vi "Stop Core.vi"(10 "final error code":i32, 11 "tWorkerTCPConnection in":refnum<class "tWorkerTCPConnection.lvclass">) -> (3 "tWorkerTCPConnection out":refnum<class "tWorkerTCPConnection.lvclass">)   [LabVIEW 2013, in "tWorkerTCPConnection.lvlib" / "tWorkerTCPConnection.lvclass"]
doc: "(<B>Filename</B>: Actor Framework.lvlib:Actor.lvclass:Stop Core.vi)\n\nDefines what the actor does before it stops. Use the <B>final error code</B> input to determine whether the actor shut down in response to an error.\n\nBy default, this method does nothing. A descendant class may override it to define behavior, such as shutting down any processes the actor initiated in its override of the Actor Core method."
uses:
  tWorkerTCPConnection.lvclass
  <vilib>/ActorFramework/Actor/Actor.lvclass
  tWorkerTCPConnection.lvclass/tWorkerTCPConnection.ctl
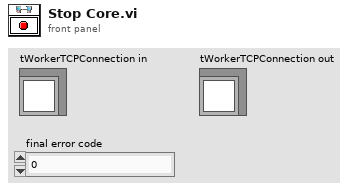
[diagram p1: front panel]
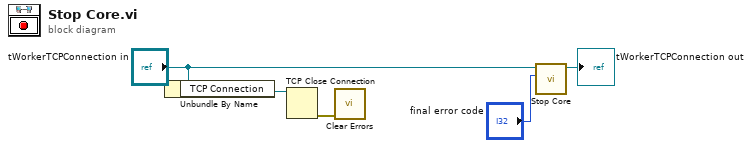
[diagram p0: block diagram]
diagram:
  n1 = Unbundle By Name("tWorkerTCPConnection in") -> ("TCP Connection"=w2:refnum<k5>)
  n2 = TCP Close Connection(connection ID=w2) -> (error out=w1:errorcluster)  [unwired: 2 in, 1 out]
  n3 = call <vilib>:"Clear Errors.vi"("error in (no error)"=w1) -> ()  [unwired: 6 in, 1 out]
  n4 = call-parent "Stop Core.vi"("final error code"="final error code", "Actor in"="tWorkerTCPConnection in") -> ("Actor out"=→"tWorkerTCPConnection out":refnum<class "tWorkerTCPConnection.lvclass">)  [unwired: 9 in]
